vi "test Pulse Width Modulation.vi"(8 "error in (no error)":errorcluster, 11 "TestCase in":refnum<class "Scan Engine cRIO System Tests.lvclass">) -> (0 "error out":errorcluster, 3 "TestCase out":refnum<class "Scan Engine cRIO System Tests.lvclass">)   [LabVIEW 2016, in "Scan Engine cRIO System Tests.lvclass"]
uses:
  Scan Engine cRIO System Tests.lvclass
  C:/Users/rzoeller/Documents/ni-official/niveristand-custom-device-testing-tools/VeriStandTestCase/VeriStandTestCase.lvclass
  <vilib>/addons/_JKI Toolkits/VI Tester/TestCase.llb/TestCase.lvclass
  niveristand-custom-device-testing-tools/VeriStandTestCase/VeriStandTestCase.lvclass
  C:/Program Files (x86)/National Instruments/LabVIEW 2016/vi.lib/addons/_JKI Toolkits/VI Tester/TestCase.llb/TestCase.lvclass
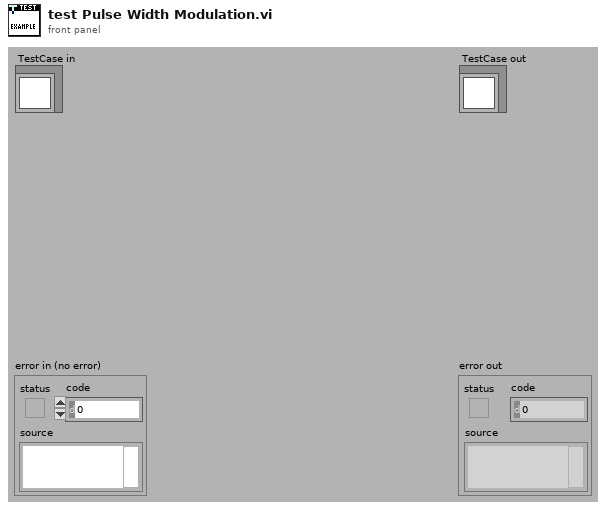
[diagram p1: front panel]
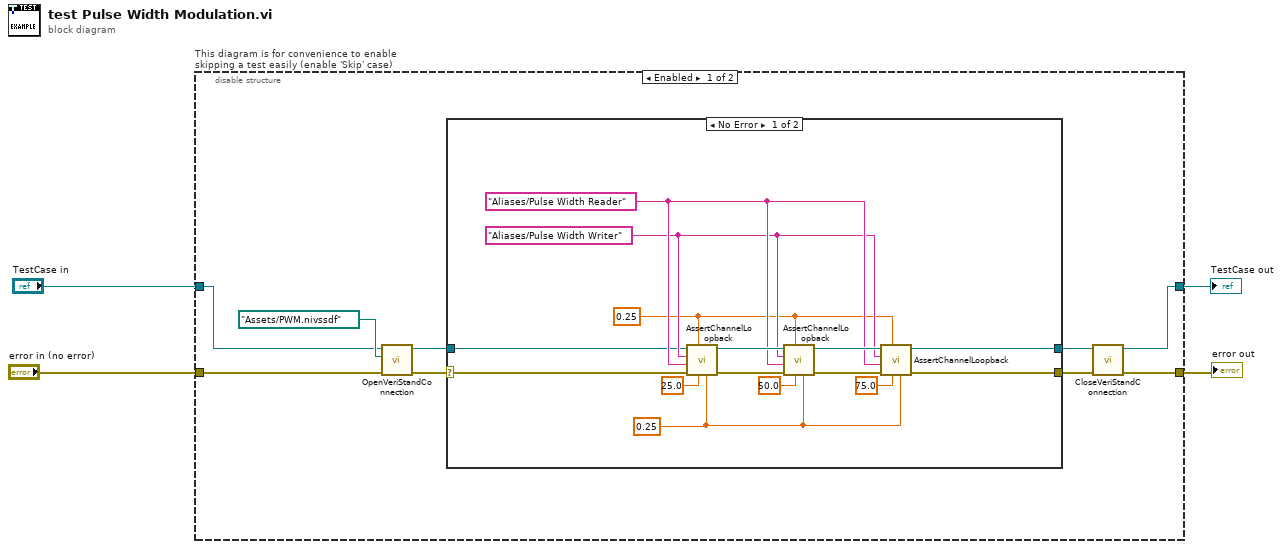
[diagram p0: block diagram]
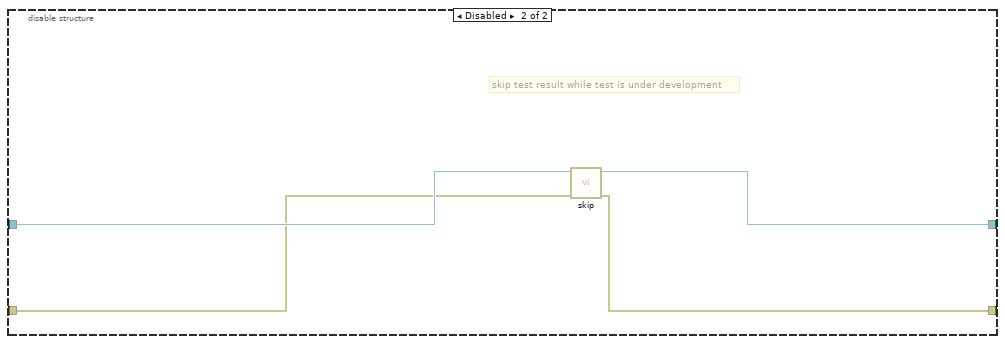
[diagram p3: hidden frame]
diagram:
  n1 = disable-structure "This diagram is for convenience to enable skipping a test easily (enable 'Skip' case)" shown="Enabled" {
    disable-tunnel: "TestCase in" -> [w9 w34]
    disable-tunnel: [w5 w32] -> w1
    disable-tunnel: [w7 w33] -> w3
    disable-tunnel: "error in (no error)" -> [w11 w31]
    frame Enabled {
      n2 = call-dynamic "OpenVeriStandConnection.vi"("error in (no error)"=w11, "System Definition File"=path "Assets/PWM.nivssdf", "VeriStand Test Case in"=w9) -> ("error out"=w12:errorcluster, "VeriStand Test Case out"=w10:refnum<class "Scan Engine cRIO System Tests.lvclass">)  [unwired: 7 in]
      n3 = case shown="No Error" w12 {
        selector: w12 -> [w14 w30]
        tunnel: [w21 w30] -> w8
        tunnel: [w23 w29] -> w6
        tunnel: w10 -> [w15 w29]
        frame No Error {
          w16 = 0.25 ("Delay Time (s)")
          w18 = 0.25 ("Tolerance")
          w19 = "Aliases/Pulse Width Writer" ("Channel")
          w20 = "Aliases/Pulse Width Reader" ("Channel")
          n4 = call "AssertChannelLoopback.vi"("Tolerance"=w18, "Value"=25.0, "Delay Time (s)"=w16, "error in (no error)"=w14, "Read Channel"=w20, "Write Channel"=w19, "VeriStand Test Case in"=w15) -> ("error out"=w26:errorcluster, "VeriStand Test Case out"=w27:refnum<class "Scan Engine cRIO System Tests.lvclass">)  [unwired: 3 in]
          n5 = call "AssertChannelLoopback.vi"("Tolerance"=w18, "Value"=50.0, "Delay Time (s)"=w16, "error in (no error)"=w26, "Read Channel"=w20, "Write Channel"=w19, "VeriStand Test Case in"=w27) -> ("error out"=w22:errorcluster, "VeriStand Test Case out"=w24:refnum<class "Scan Engine cRIO System Tests.lvclass">)  [unwired: 3 in]
          n6 = call "AssertChannelLoopback.vi"("Tolerance"=w18, "Value"=75.0, "Delay Time (s)"=w16, "error in (no error)"=w22, "Read Channel"=w20, "Write Channel"=w19, "VeriStand Test Case in"=w24) -> ("error out"=w21:errorcluster, "VeriStand Test Case out"=w23:refnum<class "Scan Engine cRIO System Tests.lvclass">)  [unwired: 3 in]
        }
        frame Error {
        }
      }
      n7 = call-dynamic "CloseVeriStandConnection.vi"("error in (no error)"=w8, "VeriStand Test Case in"=w6) -> ("error out"=w7:errorcluster, "VeriStand Test Case out"=w5:refnum<class "Scan Engine cRIO System Tests.lvclass">)  [unwired: 8 in]
    }
    frame Disabled {
      # "skip test result while test is under development"
      n8 = call <vilib>:"skip.vi"("error in (no error)"=w31, "TestCase in"=w34) -> ("error out"=w33:errorcluster, "TestCase out"=w32:refnum<class "Scan Engine cRIO System Tests.lvclass">)  [unwired: 8 in]
    }
  }
  "error out" <- w3
  "TestCase out" <- w1
